vi "Put Inside Temp Calibration Value V.vi"(8 "error in (no error)":errorcluster, 11 "calValue":sgl) -> (0 "error out":errorcluster, 3 "function return":i32)   [LabVIEW 2009, in "VantagePro.lvlib"]
doc: "DllAccess int _stdcall PutInsideTempCalibrationValue_V(float calValue);"
uses:
  VantagePro.lvlib
  <userlib>/VantagePro/VantagePro.dll
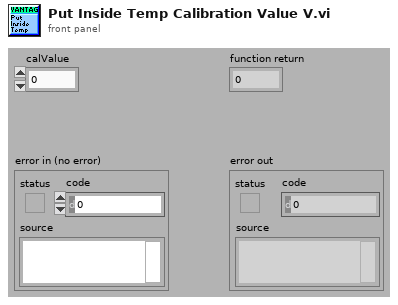
[diagram p1: front panel]
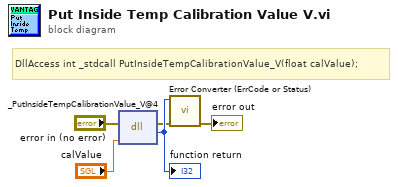
[diagram p0: block diagram]
diagram:
  # "DllAccess int _stdcall PutInsideTempCalibrationValue_V(float calValue);"
  n1 = dll-call lib="C:/Program Files/National Instruments/LabVIEW 2010/user.lib/VantagePro/VantagePro.*" fn="_PutInsideTempCalibrationValue_V@4"(error in="error in (no error)", "calValue"="calValue") -> (error out=w2:errorcluster, w5:i32)  [unwired: 3 in, 1 out]
  "function return" <- w5
  n2 = call "Error Converter (ErrCode or Status).vi"("error in (no error)"=w2, "error code"=w5) -> ("error out"=→"error out":errorcluster)  [unwired: 9 in]
